vi "placeAbove.vi"(4 "spacing":u16, 6 "useControlBodyOnly":bool, 8 "error in (no error)":errorcluster, 10 "anchorObject":refnum<vi>, 11 "movingObject":refnum<vi>) -> (0 "error out":errorcluster, 2 "anchorObject(dup)":refnum<vi>, 3 "movingObject(dup)":refnum<vi>)   [LabVIEW 2023]
doc: "Positions the 'movingObject' above the 'anchorObject' with the given spacing.\n\nThe operation affects only the Y coordinate.\nThe X coordinate of the item is not modified."
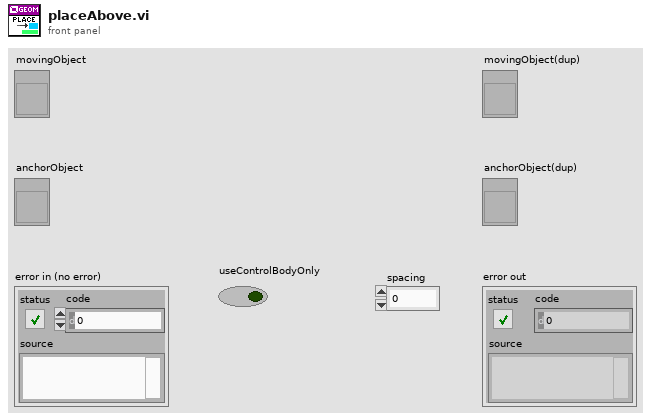
[diagram p1: front panel]
types:
  T1 = cluster{"left":i32, "top":i32, "right":i32, "bottom":i32}
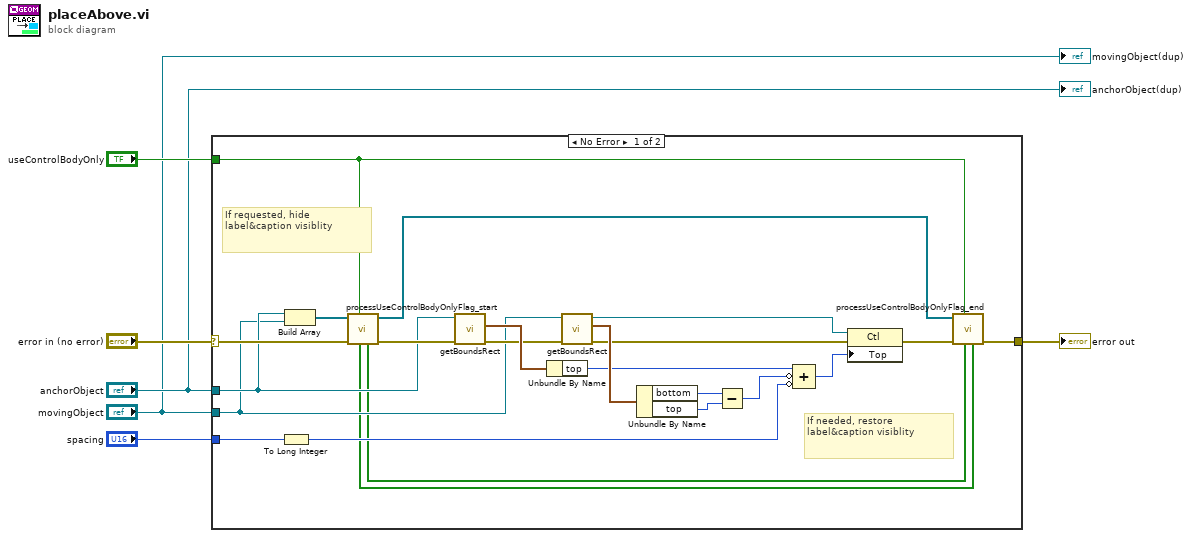
[diagram p0: block diagram]
diagram:
  n1 = case shown="No Error" "error in (no error)" {
    selector: "error in (no error)" -> [w29 w30]
    tunnel: [w26 w30] -> w6
    tunnel: "anchorObject" -> [w24 _]
    tunnel: "useControlBodyOnly" -> [w9 _]
    tunnel: "movingObject" -> [w21 _]
    tunnel: "spacing" -> [w15 _]
    frame No Error {
      # "If needed, restore label&caption visiblity"
      # "If requested, hide label&caption visiblity"
      n2 = To Long Integer(number=w15) -> (32bit integer=w14:i32)
      n3 = Build Array(w24, w21) -> (w28:refnum<vi>[])
      n4 = call "processUseControlBodyOnlyFlag_start.vi"("useControlBodyOnly"=w9, "error in (no error)"=w29, "refList"=w28) -> ("error out"=w25:errorcluster, "refList(dup)"=w27:refnum<vi>[], "LabelVisibilityList"=w8:bool[], "captionVisibilityList"=w7:bool[])  [unwired: 5 in]
      n5 = call "getBoundsRect.vi"("error in (no error)"=w25, "ref"=w24) -> ("error out"=w22:errorcluster, "rect"=w23:T1)  [unwired: 7 in, 1 out]
      n6 = Unbundle By Name(w23) -> ("top"=w18:i32)
      n7 = call "getBoundsRect.vi"("error in (no error)"=w22, "ref"=w21) -> ("error out"=w12:errorcluster, "rect"=w20:T1, "ref(dup)"=w13:refnum<vi>)  [unwired: 7 in]
      n8 = Unbundle By Name(w20) -> ("bottom"=w16:i32, "top"=w19:i32)
      n9 = Subtract(x=w16, y=w19) -> (x-y=w17:i32)
      n10 = Compound Arithmetic op=ADD(w18, invert w17, invert w14) -> (w10:i32)
      n11 = property class="Ctl"(reference=w13, error in=w12, "Top"=w10) -> (error out=w11:errorcluster)  [unwired: 1 out]
      n12 = call "processUseControlBodyOnlyFlag_end.vi"("captionVisibilityList"=w7, "LabelVisibilityList"=w8, "useControlBodyOnly"=w9, "error in (no error)"=w11, "refList"=w27) -> ("error out"=w26:errorcluster)  [unwired: 5 in, 1 out]
    }
    frame Error {
    }
  }
  "error out" <- w6
  "movingObject(dup)" <- "movingObject"
  "anchorObject(dup)" <- "anchorObject"
